vi "PV ActiveLine - OffsetCorrection (TPG362).vi"(7 "W/R":bool, 8 "Fehler (Eingang)":errorcluster, 9 "Sensor 2 Set":i8(ring) items=["deactivate", "activate", "set offset and activate", "equalize to zero"], 10 "Sensor 1 Set":i8(ring) items=["deactivate", "activate", "set offset and activate", "equalize to zero"], 11 "Referenz in":refnum<visa-resource-name>) -> (0 "Cluster (Ausgang)":errorcluster, 1 "Sensor 2 Get":i8(ring) items=["deactivate", "activate", "set offset and activate", "equalize to zero"], 2 "Sensor 1 Get":i8(ring) items=["deactivate", "activate", "set offset and activate", "equalize to zero"], 3 "Referenz out":refnum<visa-resource-name>)   [LabVIEW 2013, in "PV ActiveLine.lvlib"]
doc: "OFC - Offset Correction (Linear Gauges)\n\nTransmit: OFC [,a,b]\nReceive: a,b\n\nOffset correction gauge 1,\na =\n0 –> Off (default)\n1 –> On\n2 –> Determine offset value and activate offset correction\n3 –> Adjust the zero of linear gauge\n\nOffset correction gauge 2,\nb =\n0 –> Off (default)\n1 –> On\n2 –> Determine offset value and activate offset correction\n3 –> Adjust the zero of linear gauge"
uses:
  <instrlib>/PV ActiveLine/PV ActiveLine.lvlib
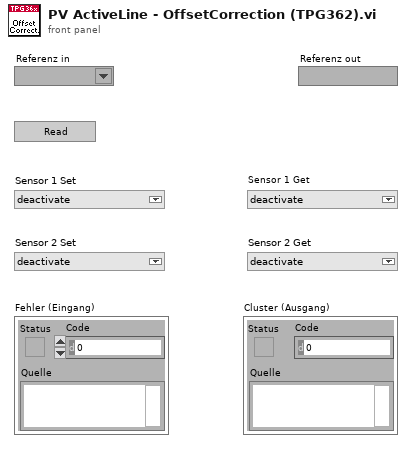
[diagram p1: front panel]
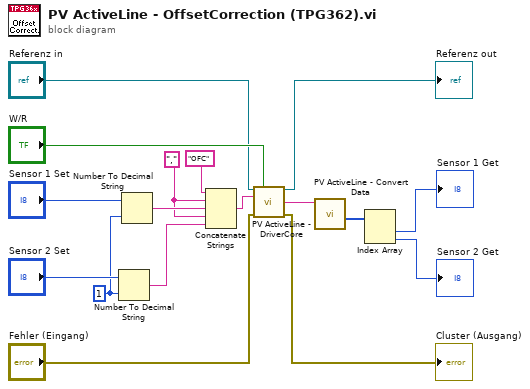
[diagram p0: block diagram]
diagram:
  w1 = i16 1 ("Breite (-)")
  w5 = "," ("Command")
  n1 = Number To Decimal String(number="Sensor 2 Set", width (-)=w1) -> (decimal integer string=w4:string)
  n2 = Number To Decimal String(number="Sensor 1 Set", width (-)=w1) -> (decimal integer string=w6:string)
  n3 = Concatenate Strings("OFC", w5, w6, w5, w4) -> (w15:string)
  n4 = call <instrlib>:"PV ActiveLine - DriverCore.vi"("Referenz in"="Referenz in", "Write/Read"="W/R", "Command"=w15, "Fehler (Eingang)"="Fehler (Eingang)") -> ("Referenz out"=→"Referenz out":refnum<visa-resource-name>, "String Out"=w10:string, "Cluster (Ausgang)"=→"Cluster (Ausgang)":errorcluster)  [unwired: 9 in]
  n5 = call <instrlib>:"PV ActiveLine - Convert Data.vi"("String in"=w10) -> ("Integer Out"=w9:i32[])  [unwired: 7 in, 3 out]
  n6 = Index Array(array=w9) -> (element #1=→"Sensor 1 Get":i32, element #2=→"Sensor 2 Get":i32)  [unwired: 2 in]
